vi "Test Enumerates Tests Starting with Verify.vi"(8 "error in (no error)":errorcluster, 11 "Test Case In":refnum<class "Test Suite Enumeration Test.lvclass">) -> (0 "error out":errorcluster, 3 "Test Case Out":refnum<class "Test Suite Enumeration Test.lvclass">)   [LabVIEW 2020, in "Test Suite Enumeration Test.lvclass"]
uses:
  Test Suite Enumeration Test.lvclass
  C:/Program Files (x86)/National Instruments/LabVIEW 2020/vi.lib/Astemes/LUnit/Core/LUnit Test Case/Test Case.lvclass
  Test Doubles/Test Case Test Double/Test Case Test Double.lvclass
  <vilib>/Astemes/LUnit/Core/LUnit Test Case/Test Case.lvclass/Test Case.ctl
  0008e1a5-151a-43f4-958d-018362b9536d.vi
  <vilib>/Astemes/LUnit/Core/LUnit Test Case/Assertions/Pass If.vi
  <vilib>/Astemes/LUnit/Core/LUnit Test Case/Private/Append Fail Result.vi
  <vilib>/Astemes/LUnit/Core/LUnit Test Case/Private/Append Pass Result.vi
  <vilib>/Astemes/LUnit/Core/LUnit Test Case/Private/Run In UI.vi
  <vilib>/Utility/error.llb/Clear Errors.vi
  source/LUnit Test Suite.lvclass
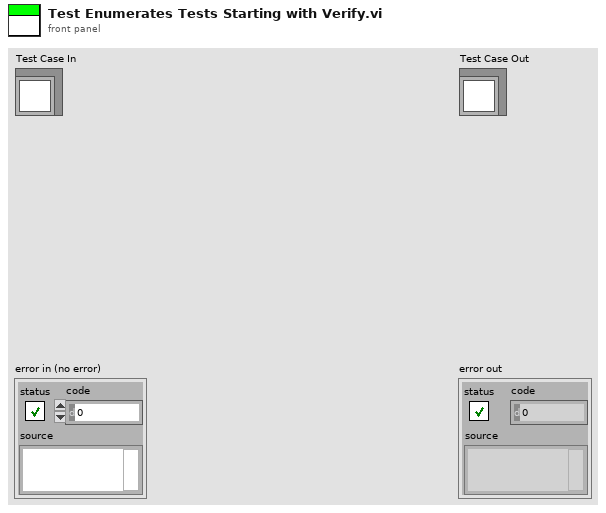
[diagram p1: front panel]
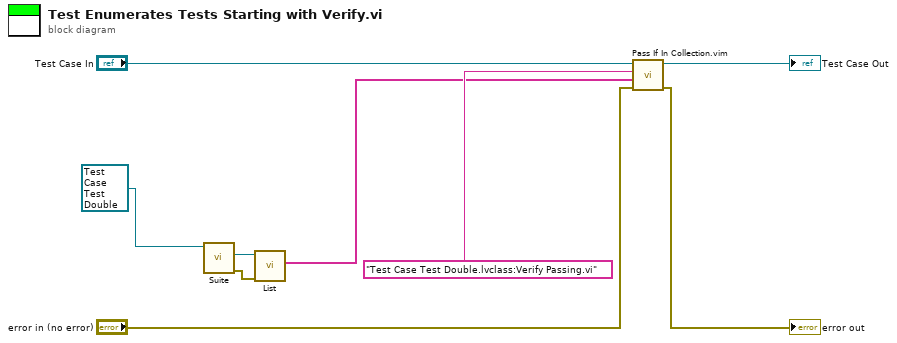
[diagram p0: block diagram]
diagram:
  n1 = call-dynamic "Suite.vi"("LUnit Test Case In"=refnum<class "Test Case Test Double.lvclass"> refnum ("Test Case Test Double.lvclass")) -> ("error out"=w4:errorcluster, "LUnit Test Suite Out"=w3:refnum<class "LUnit Test Suite.lvclass">)  [unwired: 8 in, 1 out]
  n2 = call "List.vi"("error in (no error)"=w4, "LUnit Test Suite In"=w3) -> ("List of Runnables"=w1:string[])  [unwired: 8 in, 1 out]
  n3 = call "Pass If In Collection.vim"("error in (no error)"="error in (no error)", "Collection"=w1, "Expected Element"="Test Case Test Double.lvclass:Verify Passing.vi", "LUnit Test Case In"="Test Case In") -> ("error out"=→"error out":errorcluster, "LUnit Test Case Out"=→"Test Case Out":refnum<class "Test Suite Enumeration Test.lvclass">)  [unwired: 6 in]
